vi "fetch-cluster-data-from-dbc.vi"(8 "error in (no error)":errorcluster, 11 "CLUSTER.TAG":refnum<k21>) -> (0 "error out":errorcluster, 3 "CAN Cluster":T1={"Name"="", "Baud Rate"=125000, "Application Protocol"=enum."None", "Comment"=""})   [LabVIEW 2015]
doc: "Use this template to build a VI to use as a subVI."
uses:
  controls/dbc-cluster.ctl
  <resource>/objmgr/xnet.rc
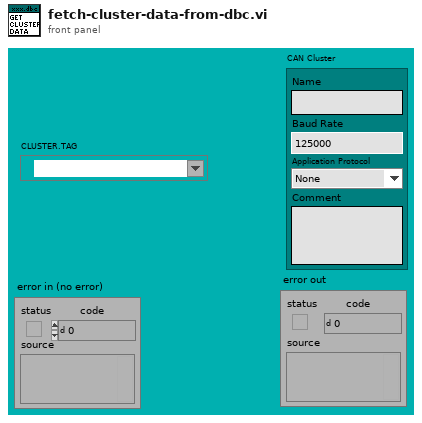
[diagram p1: front panel]
types:
  T1 = typedef "dbc-cluster.ctl" = cluster{"Name":string, "Baud Rate":u32, "Application Protocol":enum16{"None", "J1939"}, "Comment":string}
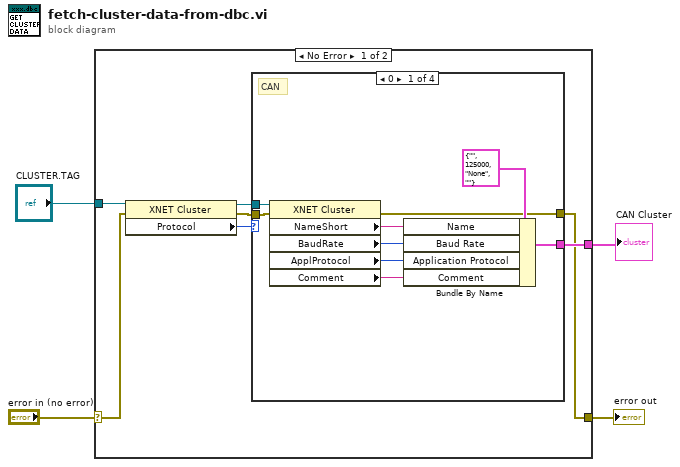
[diagram p0: block diagram]
diagram:
  n1 = case shown="No Error" "error in (no error)" {
    selector: "error in (no error)" -> [w7 w24]
    tunnel: [w6 w24] -> w3
    tunnel: "CLUSTER.TAG" -> [w5 _]
    tunnel: [w10 _] -> w1
    frame No Error {
      n2 = property class="XNET Cluster"(reference=w5, error in=w7) -> (reference out=w9:refnum<k21>, error out=w8:errorcluster, "Protocol"=w11:u32)
      n3 = case shown="0" w11 {
        tunnel: [w19 _ _ _] -> w10
        tunnel: w9 -> [w18 _ _ _]
        tunnel: w8 -> [w17 w21 w22 w23]
        tunnel: [w12 w21 w22 w23] -> w6
        frame 0 {
          # "CAN"
          n4 = property class="XNET Cluster"(reference=w18, error in=w17) -> (error out=w12:errorcluster, "NameShort"=w16:string, "BaudRate"=w15:u32, "ApplProtocol"=w13:u32, "Comment"=w14:string)  [unwired: 1 out]
          n5 = Bundle By Name(cluster=T1 {"Name"="", "Baud Rate"=125000, "Application Protocol"=enum."None", "Comment"=""} ("CAN Cluster"), "Name"=w16, "Baud Rate"=w15, "Application Protocol"=w13, "Comment"=w14) -> (w19:T1)
        }
        frame 1 {
          # "flexray"
        }
        frame 2 {
          # "LIN"
        }
        frame Default {
          # "undefined"
        }
      }
    }
    frame Error {
    }
  }
  "error out" <- w3
  "CAN Cluster" <- w1
